vi "Enqueue Message.vi"   [LabVIEW 2021, in "Architecture.lvlib" / "Message.lvclass"]
uses:
  Message.lvclass
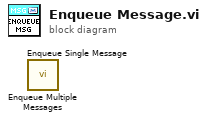
[diagram p0: block diagram]
diagram:
  n1 = call "Enqueue Multiple Messages.vi"() -> ()  [unwired: 10 in, 2 out]
  n2 = call "Enqueue Single Message.vi"() -> ()  [unwired: 10 in, 2 out]
